vi "BuildPackage.vi"(8 "error in (no error)":errorcluster, 11 "Package Builder in":refnum<class "Package Builder.lvclass">) -> (0 "error out":errorcluster, 3 "Package Builder out":refnum<class "Package Builder.lvclass">)   [LabVIEW 2020, in "Package Builder.lvclass"]
uses:
  Package Builder.lvclass
  Package Builder.lvclass/Package Builder.ctl
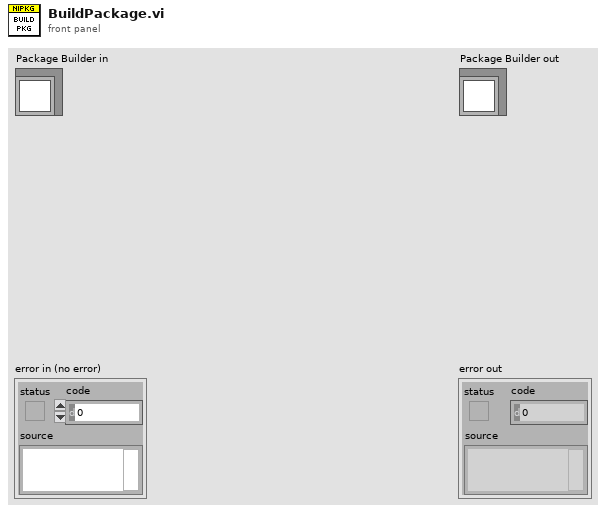
[diagram p1: front panel]
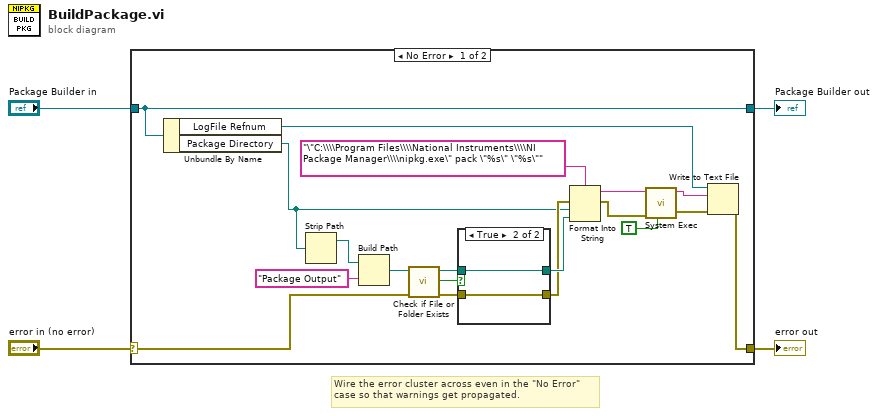
[diagram p0: block diagram]
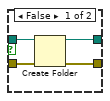
[diagram p2: hidden frame]
diagram:
  # "Wire the error cluster across even in the \"No Error\"\ncase so that warnings get propagated."
  n1 = case shown="No Error" "error in (no error)" {
    selector: "error in (no error)" -> [w8 w31]
    tunnel: [w10 w31] -> w3
    tunnel: [w15 w30] -> w1
    tunnel: "Package Builder in" -> [w15 w30]
    frame No Error {
      n2 = Unbundle By Name(w15) -> ("LogFile Refnum"=w13:refnum<file>, "Package Directory"=w14:path)
      n3 = Strip Path(path=w14) -> (stripped path=w22:path)  [unwired: 1 out]
      n4 = Build Path(base path=w22, name or relative path="Package Output" ("time format string (%c)")) -> (appended path=w9:path)
      n5 = call <vilib>:"Check if File or Folder Exists.vi"("error in (no error)"=w8, "path"=w9) -> ("error out"=w5:errorcluster, "file or folder exists?"=w6:bool, "dup path"=w7:path)  [unwired: 7 in]
      n6 = case shown="True" w6 {
        tunnel: [w27 w29] -> w18
        tunnel: [w26 w28] -> w17
        tunnel: w7 -> [w25 w29]
        tunnel: w5 -> [w24 w28]
        frame False {
          n7 = Create Folder(path (use dialog)=w25, error in=w24) -> (created path=w27:path, error out=w26:errorcluster)  [unwired: 1 in, 1 out]
        }
        frame True {
        }
      }
      n8 = Format Into String(format string="\"C:\\\\Program Files\\\\National Instruments\\\\NI Package Manager\\\\nipkg.exe\" pack \"%s\" \"%s\"" ("time format string (%c)"), error in=w17, w14, w18) -> (resulting string=w20:string, error out=w19:errorcluster)  [unwired: 1 in]
      n9 = call <vilib>:"System Exec.vi"("run minimized? (F)"=TRUE, "error in (no error)"=w19, "command line"=w20) -> ("error out"=w11:errorcluster, "standard output"=w12:string)  [unwired: 5 in, 2 out]
      n10 = Write to Text File(file (use dialog)=w13, text=w12, error in=w11) -> (error out=w10:errorcluster)  [unwired: 1 in, 2 out]
    }
    frame Error {
    }
  }
  "error out" <- w3
  "Package Builder out" <- w1
